vi "Check abort.vi"(8 "error in (no error)":errorcluster, 9 "Combine with Error (T)":bool=TRUE, 10 "Ctrl Ref in":refnum<vi>) -> (0 "error out":errorcluster, 1 "Ctrl Val":bool, 2 "Ctrl Ref out":refnum<vi>)   [LabVIEW 2018]
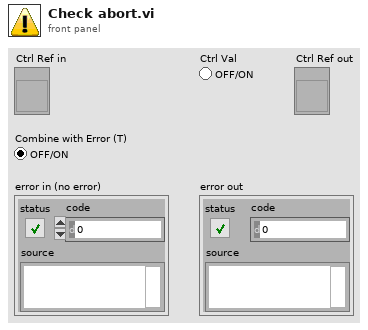
[diagram p1: front panel]
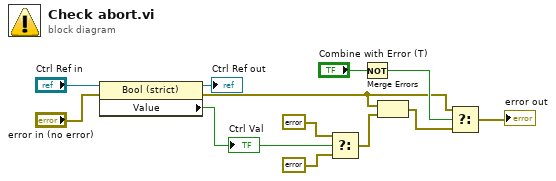
[diagram p0: block diagram]
diagram:
  n1 = property on="Property Node" class="Bool (strict)"(reference="Ctrl Ref in", error in="error in (no error)") -> (reference out=→"Ctrl Ref out":refnum<vi>, error out=w10:errorcluster, "Value"=w6:bool)
  "Ctrl Val" <- w6
  n2 = Select(t=errorcluster {"status"=TRUE, "code"=0, "source"="Abort signal received"} ("error in"), s=w6, f=errorcluster {"status"=FALSE, "code"=0, "source"=""}) -> (s? t:f=w8:errorcluster)
  n3 = Not(x="Combine with Error (T)") -> (.not. x?=w12:bool)
  n4 = Merge Errors(w10, w8) -> (w9:errorcluster)
  n5 = Select(t=w10, s=w12, f=w9) -> (s? t:f=→"error out":errorcluster)
